vi "C4Buf_getPixelformatName.vi"(0 "c4buf in":refnum<k24>, 5 "pixelformat in":i64, 11 "error in (no error)":errorcluster) -> (4 "c4buf out":refnum<k24>, 6 "pixelformatName out":string, 15 "error out":errorcluster)   [LabVIEW 2015, in "libC4HdlLV.lvlib"]
uses:
  libC4HdlLV.lvlib
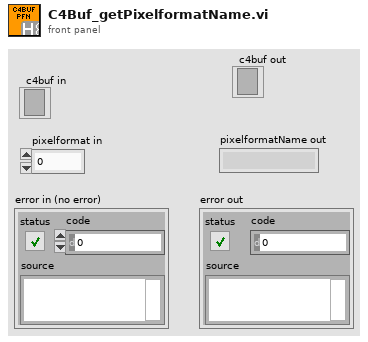
[diagram p1: front panel]
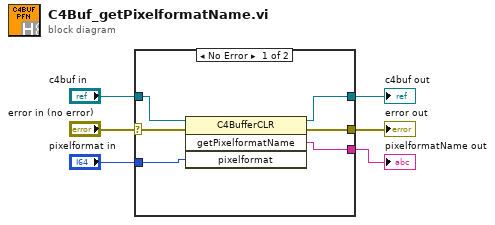
[diagram p0: block diagram]
diagram:
  n1 = case shown="No Error" "error in (no error)" {
    selector: "error in (no error)" -> [w11 w14]
    tunnel: [w10 w14] -> w5
    tunnel: "c4buf in" -> [w12 w13]
    tunnel: [w9 w13] -> w3
    tunnel: "pixelformat in" -> [w8 _]
    tunnel: [w7 _] -> w1
    frame No Error {
      n2 = invoke class="C4BufferCLR" method="getPixelformatName"(reference=w12, error in=w11, "pixelformat"=w8) -> (reference out=w9:refnum<k24>, error out=w10:errorcluster, "getPixelformatName"=w7:string)  [unwired: 1 in, 1 out]
    }
    frame Error {
    }
  }
  "error out" <- w5
  "c4buf out" <- w3
  "pixelformatName out" <- w1
